vi "F710_offline.vi"() -> ()   [LabVIEW 2019]
uses:
  <vilib>/Instr/_visa.llb/Select Event Type.ctl
panel:
  out "RT":bool
  in  "Boolean":bool
  out "Array":dbl[](array[numeric])
  out "RT":u8
  out "LT":u8
  out "RB":bool
  out "LB":bool
  out "START":bool
  out "BACK":bool
  out "X":bool
  out "B":bool
  out "A":bool
  out "Y":bool
  out "U":bool
  out "D":bool
  out "R":bool
  out "L":bool
  out "RV":i16
  out "RH":i16
  out "LV":i16
  out "(LH)":i16
  out "data buffer":u8[](array[numeric])
  out "error out":errorcluster
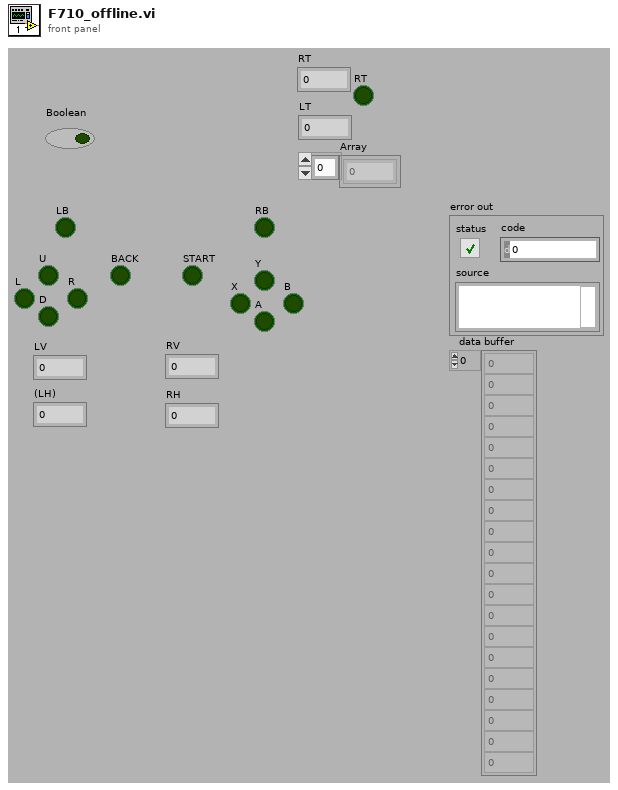
[diagram p1: front panel]
types:
  T1 = typedef "Select Event Type.ctl" = u32
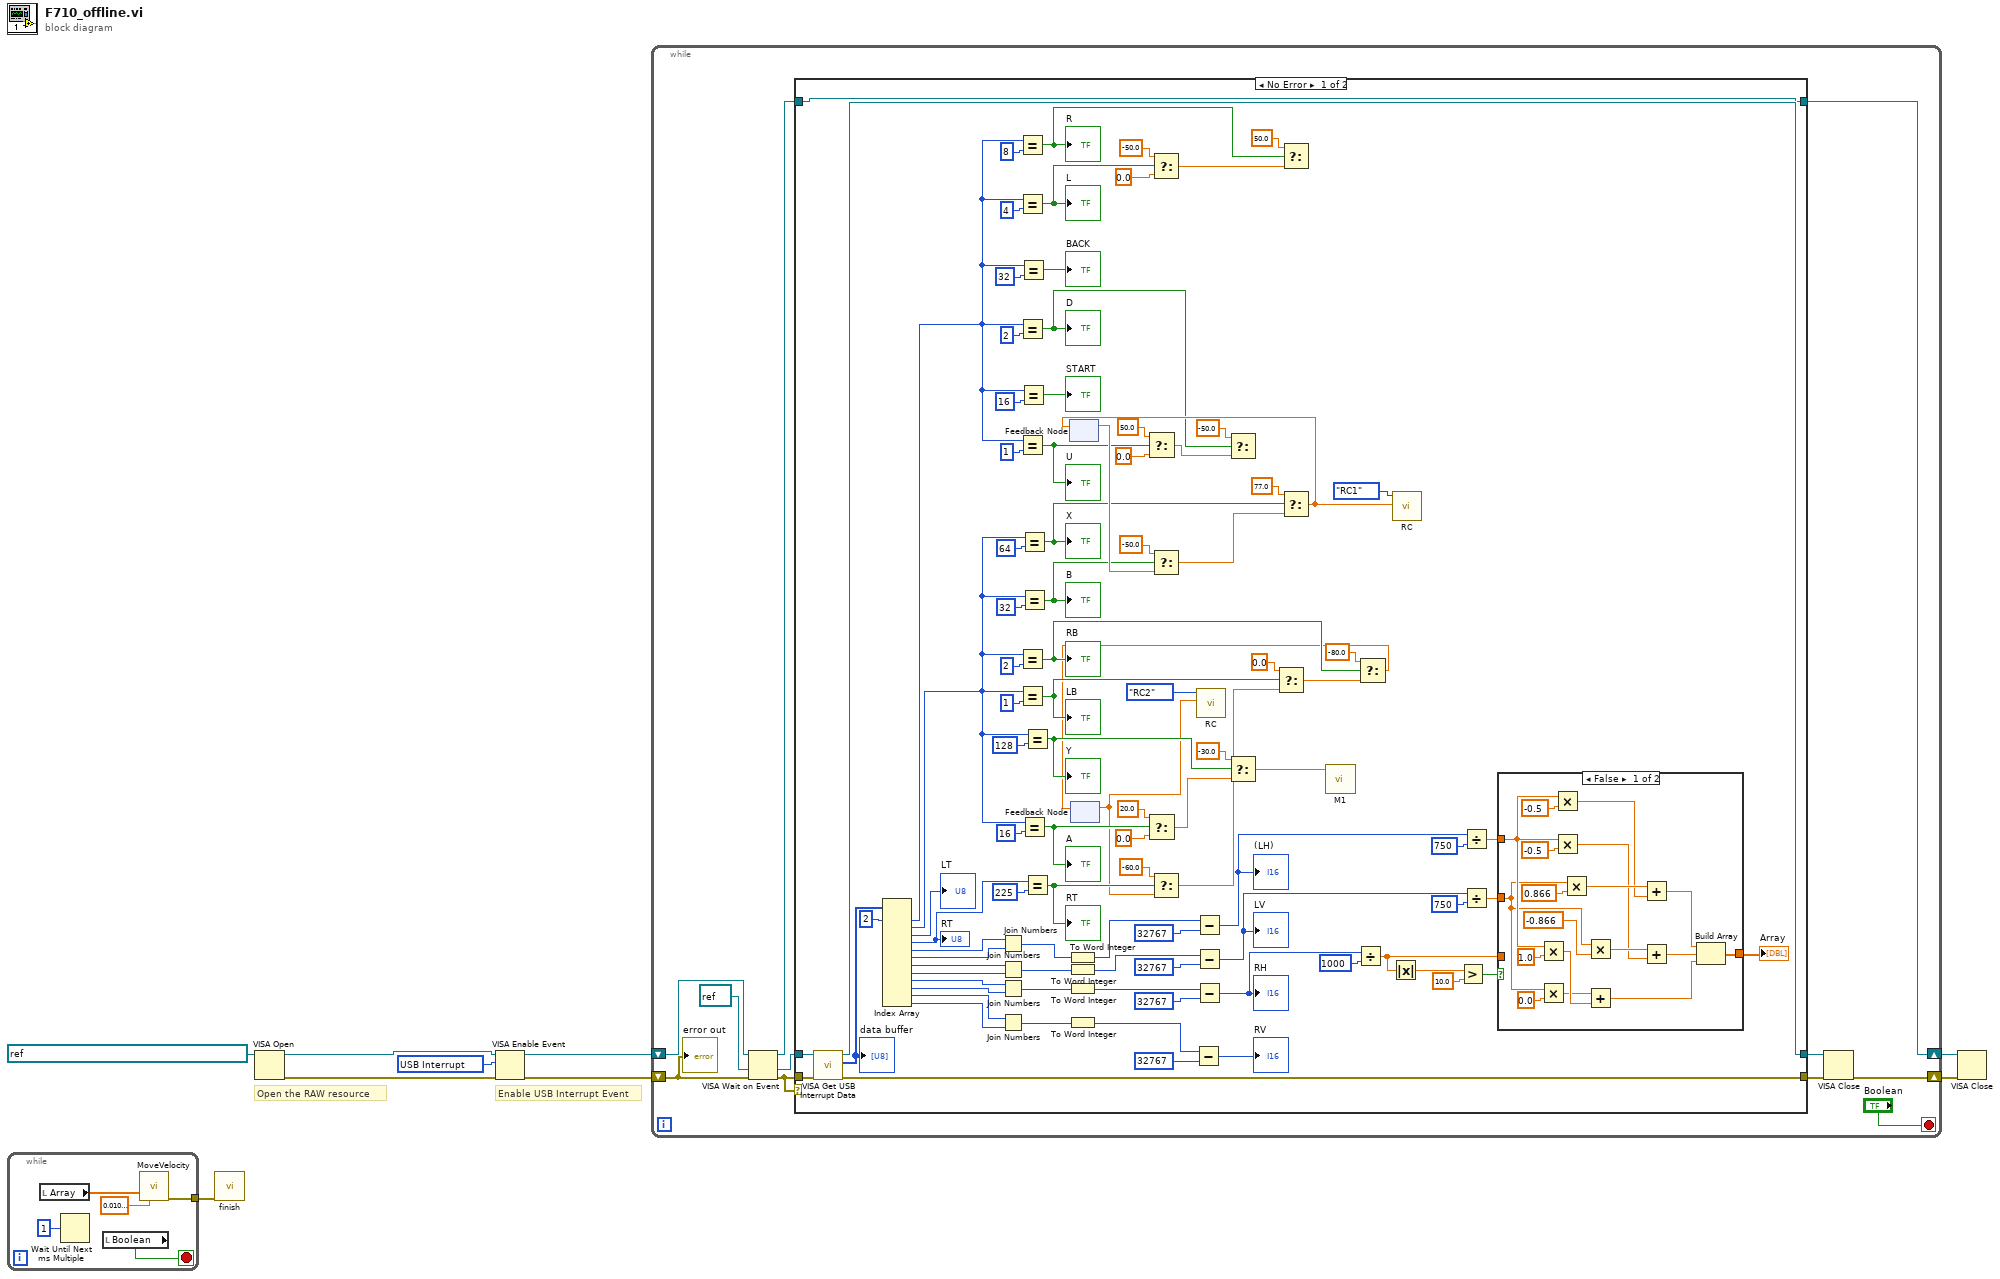
[diagram p0: block diagram]
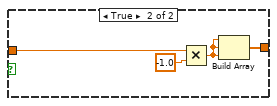
[diagram p2: hidden frame]
diagram:
  w3 = T1 1073684535 items=["Service Request"=1073684491, "Trigger"=3221168138, "Clear"=1073684493, "VXI Signal"=1073684512, "VXI/VME Interrupt"=3221168161, "VXI/VME Sysfail"=1073684509, "VXI/VME Sysreset"=1073684510, "GPIB CIC"=1073684498, "GPIB Talk"=1073684499, "GPIB Listen"=1073684500, "PXI Interrupt"=1073684514, "Serial Break"=1073684515, "Serial TermChar"=1073684516, "Serial CTS"=1073684521, "Serial DSR"=1073684522, "Serial DCD"=1073684524, "Serial RI"=1073684526, "Serial Character"=1073684533, "USB Interrupt"=1073684535, "All Enabled"=1073709055] ("Event Type")
  # "Open the RAW resource"
  # "Enable USB Interrupt Event"
  n1 = while {
    tunnel: [w13] -> w1
    stop <- w10 stop-if-true
    n2 = local read "Array"() -> (w12:dbl[])
    n3 = Wait Until Next ms Multiple(millisecond multiple=u32 1) -> ()  [unwired: 1 out]
    n4 = local read "Boolean"() -> (w10:bool)
    n5 = call "MoveVelocity.vi"("OBJ"=w12, "dt (s)"=0.010000000000000002) -> ("error out"=w13:errorcluster)  [unwired: 10 in, 3 out]
  }
  n6 = call "finish.vi"("Error/Flow In"=w1) -> ()  [unwired: 11 in]
  n7 = VISA Open(VISA resource name=refnum<visa-resource-name> "USB0::0x046D::0xC21F::AC1491AB::RAW") -> (VISA resource name=w9:refnum<visa-resource-name>, error out=w7:errorcluster)  [unwired: 1 in, 3 out]
  n8 = VISA Enable Event(8:w7, 10:w3, 11:w9) -> (0:w6:errorcluster, 3:w8:refnum<visa-resource-name>)  [unwired: 1 out]
  n9 = while {
    shift-right: [w19] -> w5
    shift-left: w8 -> [w25]
    shift-right: [w17] -> w4
    shift-left: w6 -> [w24]
    stop <- "Boolean" stop-if-true
    n10 = VISA Wait on Event(8:w24, 9:refnum<visa-resource-name> refnum ("event resource class"), 11:w25) -> (0:w21:errorcluster, 1:w23:refnum<visa-resource-name>, 3:w20:refnum<visa-resource-name>)  [unwired: 1 in, 2 out]
    n11 = case shown="No Error" w21 {
      tunnel: w23 -> [w123 w147]
      tunnel: w21 -> [w122 _]
      tunnel: [w119 _] -> w18
      tunnel: [w121 w147] -> w16
      tunnel: w20 -> [w120 w146]
      tunnel: [w120 w146] -> w19
      frame No Error {
        n12 = call <vilib>:"VISA Get USB Interrupt Data.vi"("error in (no error)"=w122, "VISA USB Intr Event"=w123) -> ("error out"=w119:errorcluster, "data buffer"=w118:u8[], "VISA USB Intr Event out"=w121:refnum<visa-resource-name>)  [unwired: 7 in]
        "data buffer" <- w118
        n13 = Index Array(array=w118, index #1=2 ("index")) -> (element #1=w83:u8, element #2=w80:u8, element #3=→"LT":u8, element #4=w32:u8, element #5=w103:u8, element #6=w102:u8, element #7=w101:u8, element #8=w100:u8, element #9=w99:u8, element #10=w98:u8, element #11=w97:u8, element #12=w96:u8)  [unwired: 11 in]
        "RT" <- w32
        n14 = Join Numbers(hi=w103, lo=w102) -> ((hi.lo)=w116:u16)
        n15 = Join Numbers(hi=w101, lo=w100) -> ((hi.lo)=w112:u16)
        n16 = Join Numbers(hi=w99, lo=w98) -> ((hi.lo)=w110:u16)
        n17 = Join Numbers(hi=w97, lo=w96) -> ((hi.lo)=w106:u16)
        n18 = Equal?(x=w83, y=u8 8) -> (x = y?=w48:bool)
        "R" <- w48
        n19 = Equal?(x=w83, y=u8 4) -> (x = y?=w52:bool)
        "L" <- w52
        n20 = Equal?(x=w83, y=u8 2) -> (x = y?=w55:bool)
        "D" <- w55
        n21 = Equal?(x=w83, y=u8 1) -> (x = y?=w58:bool)
        "U" <- w58
        n22 = Equal?(x=w80, y=u8 2) -> (x = y?=w33:bool)
        "RB" <- w33
        n23 = Equal?(x=w80, y=u8 1) -> (x = y?=w34:bool)
        "LB" <- w34
        n24 = Equal?(x=w83, y=u8 32) -> (x = y?=→"BACK":bool)
        n25 = Equal?(x=w83, y=u8 16) -> (x = y?=→"START":bool)
        n26 = Equal?(x=w80, y=u8 64) -> (x = y?=w37:bool)
        "X" <- w37
        n27 = Equal?(x=w80, y=u8 32) -> (x = y?=w38:bool)
        "B" <- w38
        n28 = Equal?(x=w80, y=u8 16) -> (x = y?=w39:bool)
        "A" <- w39
        n29 = Equal?(x=w80, y=u8 128) -> (x = y?=w35:bool)
        "Y" <- w35
        n30 = Equal?(x=w32, y=u8 225) -> (x = y?=w30:bool)
        "RT" <- w30
        n31 = To Word Integer(number=w116) -> (16bit integer=w115:i16)
        n32 = To Word Integer(number=w112) -> (16bit integer=w113:i16)
        n33 = To Word Integer(number=w110) -> (16bit integer=w109:i16)
        n34 = To Word Integer(number=w106) -> (16bit integer=w107:i16)
        n35 = feedback #1() -> (w72:dbl)  [unwired: 1 in]
        n36 = feedback #2() -> (w26:dbl)  [unwired: 1 in]
        n37 = Select(t=50.0, s=w58, f=0.0) -> (s? t:f=w56:dbl)
        n38 = Select(t=20.0, s=w39, f=0.0) -> (s? t:f=w69:dbl)
        n39 = Select(t=-50.0, s=w52, f=0.0) -> (s? t:f=w49:dbl)
        n40 = Select(t=-50.0, s=w38, f=w72) -> (s? t:f=w71:dbl)
        n41 = Select(t=-60.0, s=w30, f=w26) -> (s? t:f=w29:dbl)
        n42 = Subtract(x=w107, y=i16 32767) -> (x-y=→"RV":i16)
        n43 = Subtract(x=w115, y=i16 32767) -> (x-y=w45:i16)
        "(LH)" <- w45
        n44 = Subtract(x=w113, y=i16 32767) -> (x-y=w44:i16)
        "LV" <- w44
        n45 = Subtract(x=w109, y=i16 32767) -> (x-y=w63:i16)
        "RH" <- w63
        n46 = call "RC.vi"("數值"=w26, "選擇RC"=enum16{"請選擇RC", "RC1", "RC2", "RC3"}."RC2") -> ()  [unwired: 9 in, 1 out]
        n47 = Select(t=-50.0, s=w55, f=w56) -> ()  [unwired: 1 out]
        n48 = Select(t=-30.0, s=w35, f=w69) -> (s? t:f=w65:dbl)
        n49 = Select(t=0.0, s=w34, f=w29) -> (s? t:f=w28:dbl)
        n50 = Select(t=50.0, s=w48, f=w49) -> ()  [unwired: 1 out]
        n51 = Select(t=77.0, s=w37, f=w71) -> (s? t:f=w70:dbl)
        n52 = feedback-in #1(w70) -> ()
        n53 = call "M1.vi"("output"=w65) -> ()  [unwired: 10 in, 1 out]
        n54 = Divide(x=w63, y=i16 1000) -> (x/y=w59:dbl)
        n55 = Select(t=-80.0, s=w33, f=w28) -> (s? t:f=w27:dbl)
        n56 = feedback-in #2(w27) -> ()
        n57 = Absolute Value(x=w59) -> (abs(x)=w62:dbl)
        n58 = call "RC.vi"("數值"=w70, "選擇RC"=enum16{"請選擇RC", "RC1", "RC2", "RC3"}."RC1") -> ()  [unwired: 9 in, 1 out]
        n59 = Greater?(x=w62, y=10.0) -> (0:w60:bool)
        n60 = Divide(x=w45, y=i16 750) -> (x/y=w41:dbl)
        n61 = Divide(x=w44, y=i16 750) -> (x/y=w40:dbl)
        n62 = case shown="False" w60 {
          tunnel: w59 -> [_ w143]
          tunnel: w40 -> [w125 _]
          tunnel: w41 -> [w126 _]
          tunnel: [w124 w142] -> w46
          frame False {
            n63 = Multiply(x=w126, y=1.0) -> (x*y=w131:dbl)
            n64 = Multiply(x=w125, y=0.0) -> (x*y=w130:dbl)
            n65 = Multiply(x=w126, y=-0.5) -> (x*y=w138:dbl)
            n66 = Multiply(x=w126, y=-0.5) -> (x*y=w134:dbl)
            n67 = Multiply(x=w125, y=0.866) -> (x*y=w139:dbl)
            n68 = Multiply(x=w125, y=-0.866) -> (x*y=w135:dbl)
            n69 = Add(x=w130, y=w131) -> (x+y=w127:dbl)
            n70 = Add(x=w139, y=w138) -> (x+y=w129:dbl)
            n71 = Add(x=w135, y=w134) -> (x+y=w128:dbl)
            n72 = Build Array(w129, w128, w127) -> (w124:dbl[])
          }
          frame True {
            n73 = Multiply(x=w143, y=-1.0) -> (x*y=w144:dbl)
            n74 = Build Array(w144, w144, w144) -> (w142:dbl[])
          }
        }
        "Array" <- w46
      }
      frame Error {
      }
    }
    n75 = VISA Close(VISA resource name=w16, error in (no error)=w18) -> (error out=w17:errorcluster)
    "error out" <- w24
  }
  n76 = VISA Close(VISA resource name=w5, error in (no error)=w4) -> ()  [unwired: 1 out]
